vi "Acquire Signal.vi"(8 "error in":errorcluster, 9 "timeout":dbl=10.0 format="%0.2f", 10 "number of samples per channel":i32=-1, 11 "task/channels in":refnum<k21>) -> (0 "error out":errorcluster, 2 "data":waveform(dbl), 3 "task out":refnum<k21>)   [LabVIEW 2018]
doc: "Rejestracja sygnału napięciowego na wybranym kanale karty DAQ."
uses:
  <vilib>/DAQmx/read.llb/DAQmx Read (Analog Wfm 1Chan NSamp).vi
  <vilib>/DAQmx/miscellaneous.llb/DAQmx Fill In Error Info.vi
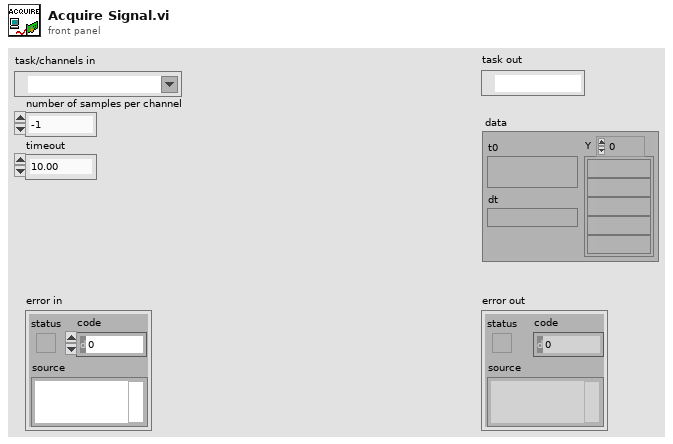
[diagram p1: front panel]
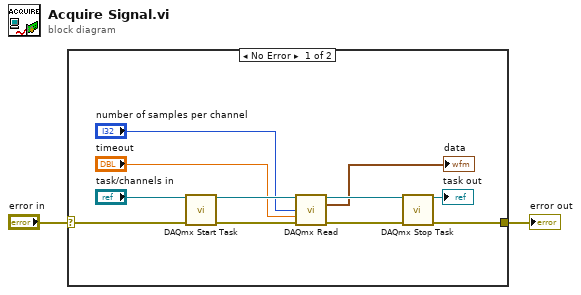
[diagram p0: block diagram]
diagram:
  n1 = case shown="No Error" "error in" {
    selector: "error in" -> [w4 w14]
    tunnel: [w9 w14] -> w2
    frame No Error {
      n2 = call <vilib>:"DAQmx Start Task.vi"("task/channels in"="task/channels in", "error in"=w4) -> ("task out"=w10:refnum<k21>, "error out"=w13:errorcluster)  [unwired: 12 in]
      n3 = call-poly <vilib>:"DAQmx Read.vi"("task/channels in"=w10, "number of samples per channel"="number of samples per channel", "timeout"="timeout", "error in"=w13) -> ("task out"=w11:refnum<k21>, "data"=→"data":waveform(dbl), "error out"=w12:errorcluster)  [unwired: 9 in]
      n4 = call <vilib>:"DAQmx Stop Task.vi"("task/channels in"=w11, "error in"=w12) -> ("task out"=→"task out":refnum<k21>, "error out"=w9:errorcluster)  [unwired: 12 in]
    }
    frame Error {
    }
  }
  "error out" <- w2
